vi "Get Step Alias Names.vi"(10 "Properties:Main Steps":refnum<class "Step Config.lvclass">[](array[class])) -> (2 "Steps Alias":string[](array[string]))   [LabVIEW 2015, in "Sequence Config.lvclass"]
uses:
  Sequence Config.lvclass
  Step/Config/Step Config.lvclass
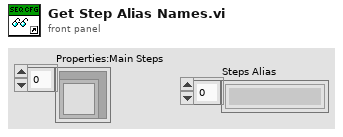
[diagram p1: front panel]
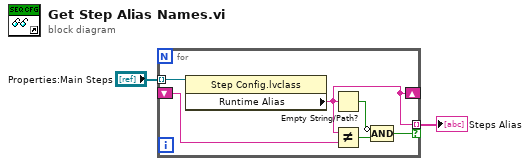
[diagram p0: block diagram]
diagram:
  n1 = for {
    tunnel: "Properties:Main Steps" -> [w8] mode=indexing
    shift-right: [w5] -> _
    shift-left: _ -> [w7]
    tunnel: [w5] -> w1 mode=indexing if=w4
    n2 = property class="Step Config.lvclass"(reference=w8) -> ("Runtime Alias"=w5:string)  [unwired: 1 in, 2 out]
    n3 = Empty String/Path?(string/path=w5) -> (empty?=w3:bool)
    n4 = Not Equal?(x=w5, y=w7) -> (x != y?=w6:bool)
    n5 = Compound Arithmetic op=AND(invert w3, w6) -> (w4:bool)
  }
  "Steps Alias" <- w1
